vi "CallRosco.vi"(6 "StopLV":bool, 8 "error in (no error)":errorcluster, 9 "ROSCO Params in":T3, 10 "Index In":T1={"iSTATUS"=0, "TIME"=1, "DT"=2, "BL_PITCH_1"=3, "VS_MECHGENPWR"=13, "GEN_SPEED"=19, "ROT_SPEED"=20, "GENTQMEAS"=22, "Y_M"=23, "HORWINDV"=26, "ROOTMOOP1"=29, "ROOTMOOP2"=30, "BL_PITCH_2"=32, "BL_PITCH_3"=33, "ROOTMOOP3"=31, "INFILE_SIZE"=49, "FA_ACC"=52, "NUM_BLADES"=60, " OUT BL_PITCH"=44, "OUT_ TORQUE"=46, "OUTFILE_SIZE "=50, "AVCMSG_SIZE"=48, "AERODYN TQ"=89, "VS_GENPWR"=14}, 11 "SwapIn":T2) -> (0 "error out":errorcluster, 1 "ROSCO Params out":T3, 2 "IndexOut":T1={"iSTATUS"=0, "TIME"=1, "DT"=2, "BL_PITCH_1"=3, "VS_MECHGENPWR"=13, "GEN_SPEED"=19, "ROT_SPEED"=20, "GENTQMEAS"=22, "Y_M"=23, "HORWINDV"=26, "ROOTMOOP1"=29, "ROOTMOOP2"=30, "BL_PITCH_2"=32, "BL_PITCH_3"=33, "ROOTMOOP3"=31, "INFILE_SIZE"=49, "FA_ACC"=52, "NUM_BLADES"=60, " OUT BL_PITCH"=44, "OUT_ TORQUE"=46, "OUTFILE_SIZE "=49, "AVCMSG_SIZE"=49, "AERODYN TQ"=46, "VS_GENPWR"=13}, 3 "SwapOut":T2)   [LabVIEW 2018]
uses:
  Clusters/RoscoParams.ctl
  Clusters/SwapIn.ctl
  Clusters/SwapIndexes.ctl
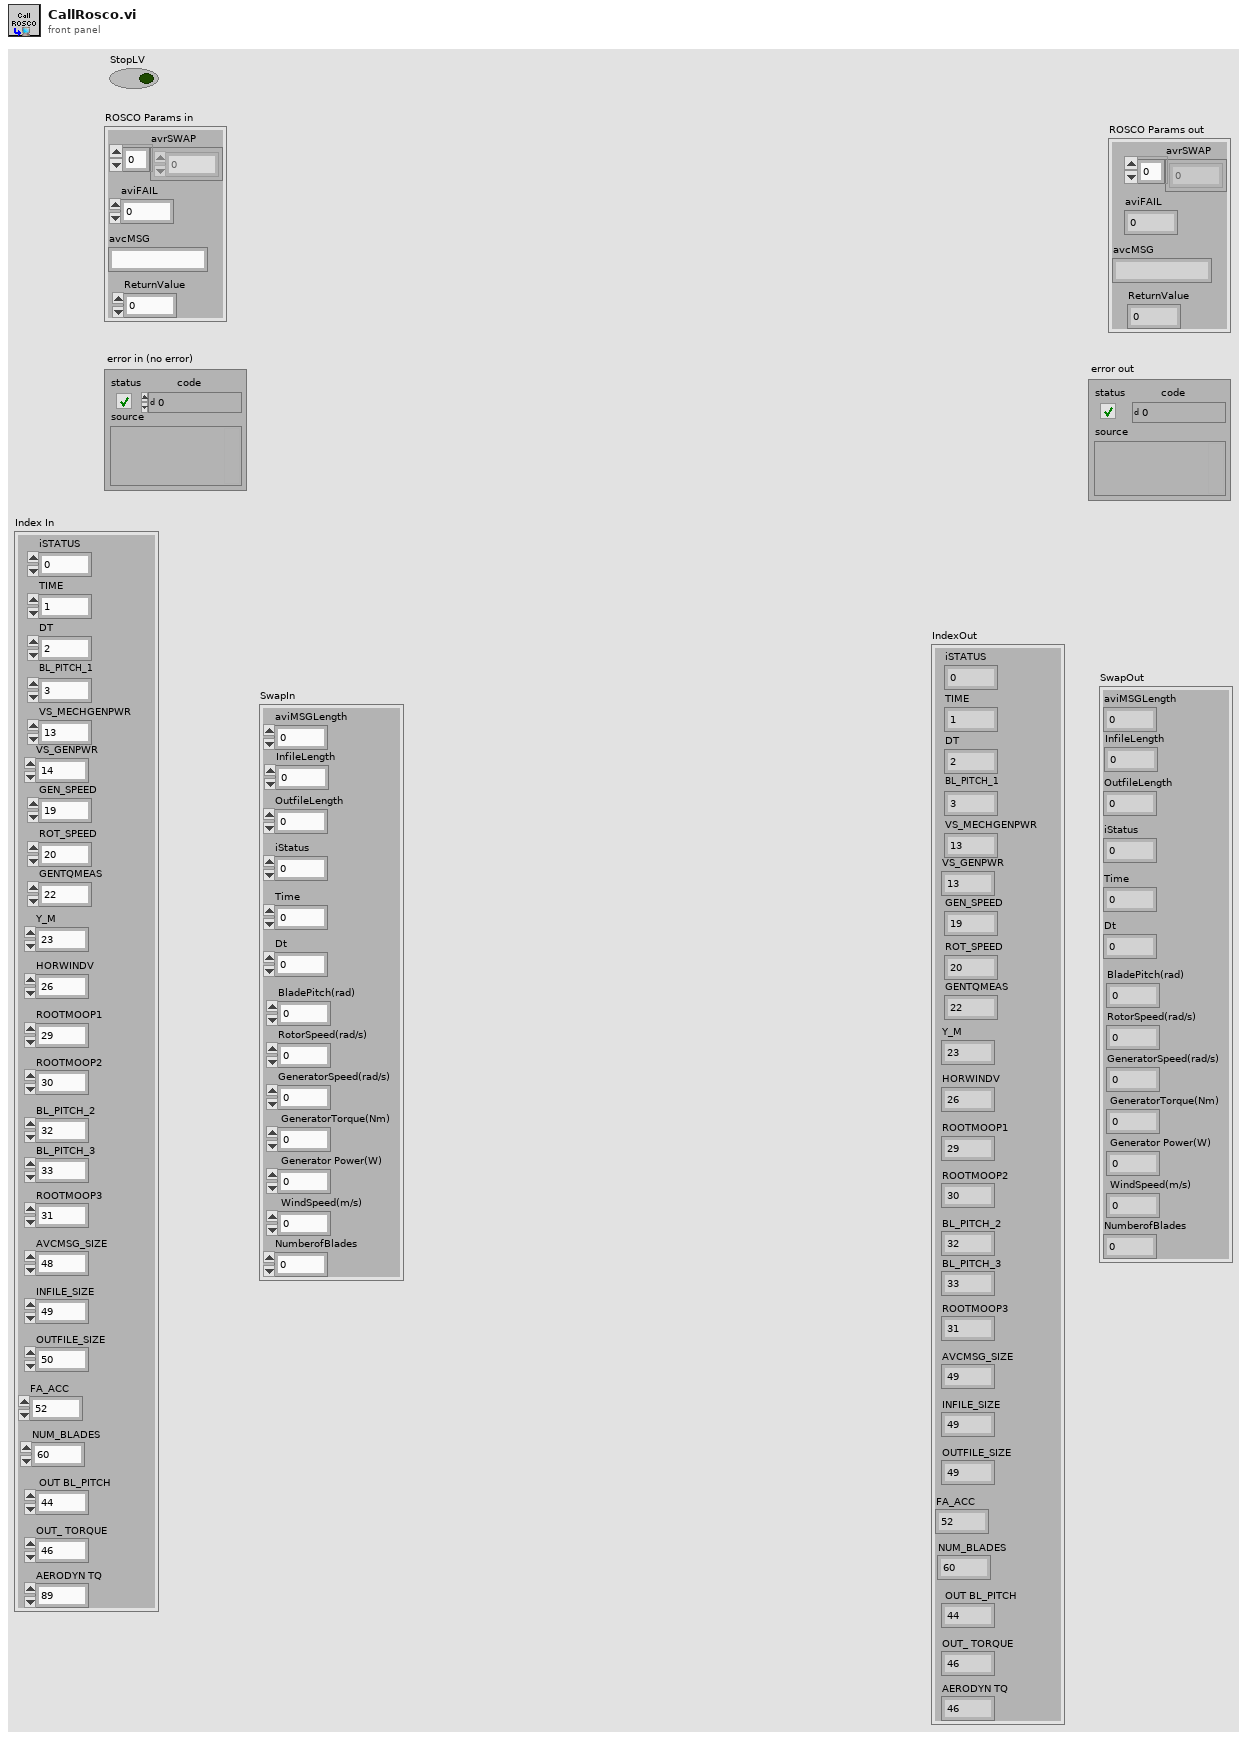
[diagram p1: front panel]
types:
  T1 = typedef "SwapIndexes.ctl" = cluster{"iSTATUS":i32, "TIME":i32, "DT":i32, "BL_PITCH_1":i32, "VS_MECHGENPWR":i32, "GEN_SPEED":i32, "ROT_SPEED":i32, "GENTQMEAS":i32, "Y_M":i32, "HORWINDV":i32, "ROOTMOOP1":i32, "ROOTMOOP2":i32, "BL_PITCH_2":i32, "BL_PITCH_3":i32, "ROOTMOOP3":i32, "INFILE_SIZE":i32, "FA_ACC":i32, "NUM_BLADES":i32, " OUT BL_PITCH":i32, "OUT_ TORQUE":i32, "OUTFILE_SIZE ":i32, "AVCMSG_SIZE":i32, "AERODYN TQ":i32, "VS_GENPWR":i32}
  T2 = typedef "SwapIn.ctl" = cluster{"BladePitch(rad)":sgl, "RotorSpeed(rad/s)":sgl, "GeneratorSpeed(rad/s)":sgl, " GeneratorTorque(Nm)":sgl, " Generator Power(W) ":sgl, " WindSpeed(m/s)":sgl, "aviMSGLength":sgl, "InfileLength":sgl, "OutfileLength":sgl, "iStatus":sgl, "Time":sgl, "Dt":sgl, "NumberofBlades":sgl}
  T3 = typedef "RoscoParams.ctl" = cluster{"avrSWAP":sgl[], "aviFAIL":i32, "avcMSG":string, "ReturnValue":i32}
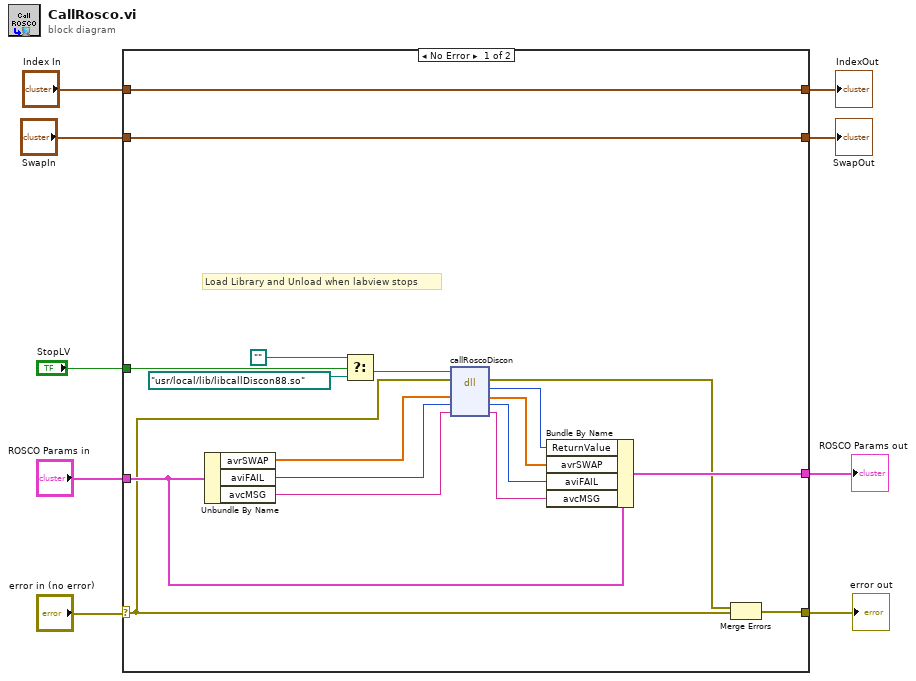
[diagram p0: block diagram]
diagram:
  n1 = case shown="No Error" "error in (no error)" {
    selector: "error in (no error)" -> [w12 w30]
    tunnel: [w26 w31] -> w9
    tunnel: "ROSCO Params in" -> [w25 w31]
    tunnel: "StopLV" -> [w22 _]
    tunnel: [w14 w30] -> w5
    tunnel: "Index In" -> [w11 w29]
    tunnel: "SwapIn" -> [w10 w28]
    tunnel: [w11 w29] -> w2
    tunnel: [w10 w28] -> w1
    frame No Error {
      # "Load Library and Unload when labview stops"
      n2 = Unbundle By Name(w25) -> ("avrSWAP"=w21:sgl[], "aviFAIL"=w19:i32, "avcMSG"=w20:string)
      n3 = Select(t=path "", s=w22, f=path "/usr/local/lib/libcallDiscon88.so") -> (s? t:f=w18:path)
      n4 = dll-call lib="usr/local/lib/callDisconTest2.so" fn="callRoscoDiscon"(path in=w18, error in=w12, "avrSWAP"=w21, "aviFAIL"=w19, "arg3avcMSG"=w20) -> (error out=w13:errorcluster, "return type"=w15:i32, "avrSWAP"=w23:sgl[], "aviFAIL"=w27:i32, "arg3avcMSG"=w24:string)  [unwired: 1 in, 1 out]
      n5 = Bundle By Name(cluster=w25, "ReturnValue"=w15, "avrSWAP"=w23, "aviFAIL"=w27, "avcMSG"=w24) -> (w26:T3)
      n6 = Merge Errors(w13, w12) -> (w14:errorcluster)
    }
    frame Error {
    }
  }
  "ROSCO Params out" <- w9
  "error out" <- w5
  "SwapOut" <- w1
  "IndexOut" <- w2
